vi "Send Message.vi"(6 "priority":i32, 8 "error in (no error)":errorcluster, 9 "timeout ms (-1)":i32=-1, 10 "Message":refnum<class "Message.lvclass">, 11 "Message Stream in":refnum<class "Message Stream.lvclass">) -> (0 "error out":errorcluster, 3 "Message Stream out":refnum<class "Message Stream.lvclass">)   [LabVIEW 2020, in "Message Stream.lvclass"]
doc: "Override this method to specify the action the local copy of this object will perform to send a message to its remote counterpart."
uses:
  Message Stream.lvclass
  <vilib>/ErrorRing/Error Ring.xnode
  <vilib>/Utility/error.llb/Error Cluster From Error Code.vi
  <vilib>/ActorFramework/Message/Message.lvclass
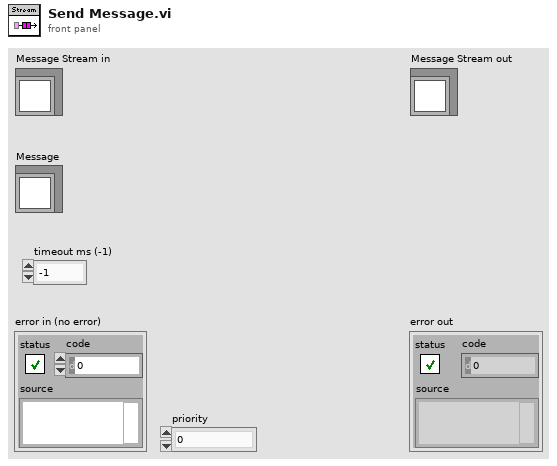
[diagram p1: front panel]
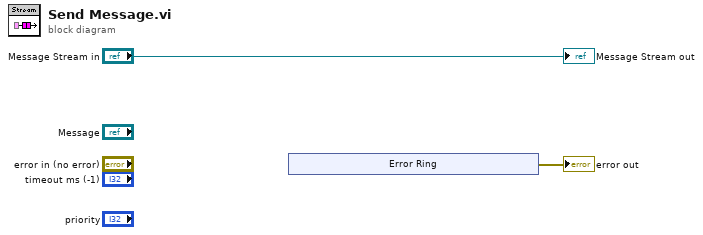
[diagram p0: block diagram]
diagram:
  n1 = xnode "Error Ring"() -> ("error out"=→"error out":errorcluster)
  "Message Stream out" <- "Message Stream in"
